vi "MenuConfig_ColorRead.vi"(8 "error in (no error)":errorcluster, 10 "Color.Name (\"Default\")":string="Default", 11 "MenuConfig":variant) -> (0 "error out":errorcluster, 2 "Colors[4]":cluster{u32, u32}[](array[cluster]), 3 "MenuConfig":variant)   [LabVIEW 2019, in "Menu Button.xctl"]
doc: "JSMA Module Template - Top Level UI 0.2.0.4\nRob Humfeld - Jet Engineering\nCopyright (c) 2019, Jet Engineering"
uses:
  Menu Button.xctl
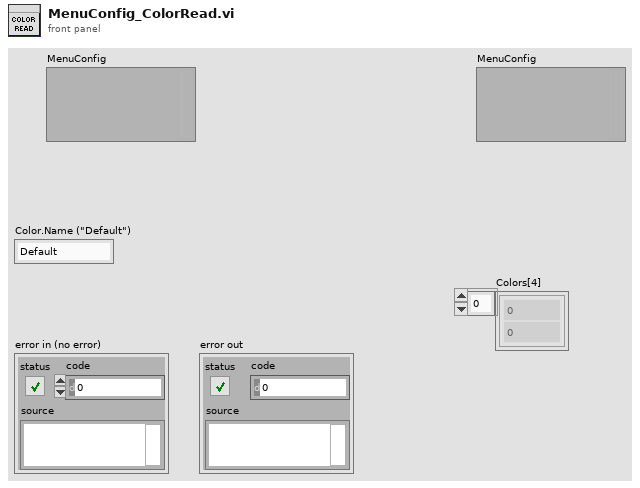
[diagram p1: front panel]
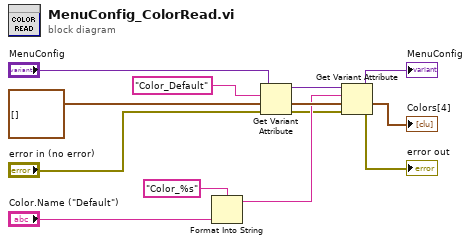
[diagram p0: block diagram]
diagram:
  n1 = Format Into String(format string="Color_%s" ("name"), "Color.Name (\"Default\")") -> (resulting string=w5:string)  [unwired: 2 in, 1 out]
  n2 = Get Variant Attribute(Variant="MenuConfig", name="Color_Default", default value (empty Variant)=cluster{u32, u32}[] [], error in="error in (no error)") -> (duplicate Variant=w9:variant, value=w6:cluster{u32, u32}[], error out=w3:errorcluster)  [unwired: 1 out]
  n3 = Get Variant Attribute(Variant=w9, name=w5, default value (empty Variant)=w6, error in=w3) -> (duplicate Variant=→"MenuConfig":variant, value=→"Colors[4]":cluster{u32, u32}[], error out=→"error out":errorcluster)  [unwired: 1 out]
